vi "FGA NL Add Node.vi"(1 "Node ID":u8, 2 "ComponentSeq":T1[](array[typedef])) -> (0 "Added?":bool)   [LabVIEW 2009]
uses:
  ComponentRec.ctl
  ServiceRec.ctl
  NodeRec.ctl
  cRIO/Functional Global Variables/Actions for FG's.ctl
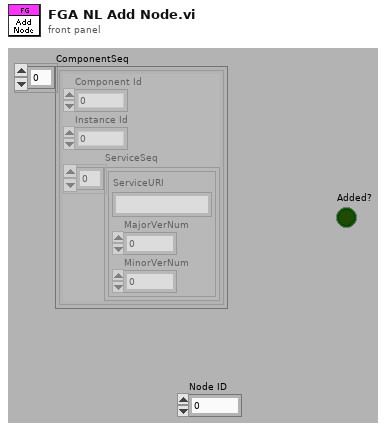
[diagram p1: front panel]
types:
  T1 = typedef "ComponentRec.ctl" = cluster{"Component Id":u8, "Instance Id":u8, "ServiceSeq":T2[]}
  T2 = typedef "ServiceRec.ctl" = cluster{"ServiceURI":string, "MajorVerNum":u8, "MinorVerNum":u8}
  T3 = typedef "NodeRec.ctl" = cluster{"Node Id":u8, "ComponentSeq":T1[]}
  T4 = typedef "Actions for FG's.ctl" = enum16{"Read", "Write"}
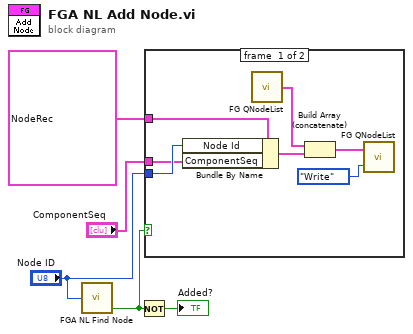
[diagram p0: block diagram]
diagram:
  n1 = call "FGA NL Find Node.vi"("Node ID"="Node ID") -> ("Record Exists?"=w3:bool)  [unwired: 2 in, 2 out]
  n2 = Not(x=w3) -> (.not. x?=→"Added?":bool)
  n3 = case shown="False" w3 {
    tunnel: T3 {"Node Id"=1, "ComponentSeq"=[{"Component Id"=1, "Instance Id"=0, "ServiceSeq"=[{"ServiceURI"="Service", "MajorVerNum"=1, "MinorVerNum"=1}]}]} ("Record out") -> [w12 _]
    tunnel: "Node ID" -> [w7 _]
    tunnel: "ComponentSeq" -> [w6 _]
    frame #0 {
      n4 = Bundle By Name(cluster=w12, "Node Id"=w7, "ComponentSeq"=w6) -> (w10:T3)
      n5 = call "FG QNodeList.vi"() -> ("NodeList out"=w11:T3[])  [unwired: 2 in]
      n6 = Build Array (concatenate)(w11, w10) -> (w9:T3[])
      n7 = call "FG QNodeList.vi"("FG Action (Read)"=Actions_for_FG's."Write", "NodeList in"=w9) -> ()  [unwired: 1 out]
    }
    frame #1 {
    }
  }
